vi "Auto Fire.vi"(11 "Run?":bool) -> (3 "Done":bool)   [LabVIEW 2013]
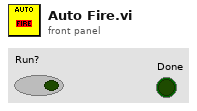
[diagram p1: front panel]
types:
  T1 = typedef "WPI_MotorControlDeviceRef.ctl" = cluster{"DeviceStatus":errorcluster, "Type":enum16{"PWM", "CAN"}, "PWM":cluster{"Digital Module":T2, "PWM Channel":T3, "DeadBand":T4}, "CAN":cluster{"Device Number":u8, "Control Mode":T5, "Semaphore":T6, "Max Vout":dbl}, "Invert":bool, "TransformRef":T7, "InvTransformRef":T7}
  T2 = typedef "FPGA_TypedefDigitalModule.ctl" = enum16{"Digital Module 1", "Digital Module 2"}
  T3 = typedef "FPGA_DIOPWMChannel.ctl" = enum8{"PWM 1", "PWM 2", "PWM 3", "PWM 4", "PWM 5", "PWM 6", "PWM 7", "PWM 8", "PWM 9", "PWM 10", "Invalid"}
  T4 = typedef "WPI_PWMDeadband.ctl" = cluster{"Name":string, "maxPositivePwm":i32, "minPositivePwm":i32, "centerPwm":i32, "maxNegativePwm":i32, "minNegativePwm":i32, "angularRange":u16}
  T5 = typedef "WPI_CANJaguar_ControlMode.ctl" = enum8{"Percent VBus", "Current", "Speed", "Position", "Voltage"}
  T6 = typedef "Semaphore RefNum" = refnum<k1>
  T7 = typedef "WPI_PWMTransform_ConPane.ctl" = refnum<vi>
  T8 = typedef "WPI_DigitalInputDevRef.ctl" = cluster{"DevStatus":errorcluster, "DIO Channel":T9, "Digital Module":T2}
  T9 = typedef "FPGA_DIOChannel.ctl" = enum8{"DIO 1", "DIO 2", "DIO 3", "DIO 4", "DIO 5", "DIO 6", "DIO 7", "DIO 8", "DIO 9", "DIO 10", "DIO 11", "DIO 12", "DIO 13", "DIO 14", "Invalid"}
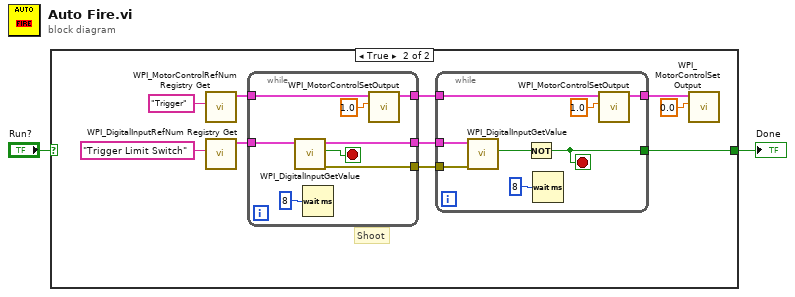
[diagram p0: block diagram]
diagram:
  n1 = case shown="True" "Run?" {
    selector: "Run?" -> [w3 _]
    tunnel: [w3 w4] -> w1
    frame False {
    }
    frame True {
      # "Shoot"
      n2 = call <vilib>:"WPI_MotorControlRefNum Registry Get.vi"("refnum name"="Trigger") -> ("MotorControlDevRef"=w10:T1)  [unwired: 9 in, 1 out]
      n3 = call <vilib>:"WPI_DigitalInputRefNum Registry Get.vi"("refnum name"="Trigger Limit Switch") -> ("DigitalInputDevRef"=w8:T8)  [unwired: 9 in, 1 out]
      n4 = while {
        tunnel: w8 -> [w21]
        tunnel: [w19] -> w5
        tunnel: [w17] -> w6
        tunnel: w10 -> [w15]
        tunnel: [w14] -> w11
        stop <- w20 stop-if-true
        n5 = call <vilib>:"WPI_DigitalInputGetValue.vi"("DigitalInputDevRef"=w21) -> ("error out"=w17:errorcluster, "Value"=w20:bool, "DigitalInputDevRef"=w19:T8)  [unwired: 8 in]
        n6 = Wait (ms)(milliseconds to wait=u32 8) -> ()  [unwired: 1 out]
        n7 = call <vilib>:"WPI_MotorControlSetOutput.vi"("Output"=1.0, "MotorControlDevRef"=w15) -> ("MotorControlDevRef"=w14:T1)  [unwired: 7 in, 2 out]
      }
      n8 = while {
        tunnel: w5 -> [w29]
        tunnel: w6 -> [w26]
        tunnel: w11 -> [w25]
        tunnel: [w23] -> w12
        tunnel: [w22] -> w4
        stop <- w22 stop-if-true
        n9 = call <vilib>:"WPI_DigitalInputGetValue.vi"("error in (no error)"=w26, "DigitalInputDevRef"=w29) -> ("Value"=w28:bool)  [unwired: 7 in, 2 out]
        n10 = Not(x=w28) -> (.not. x?=w22:bool)
        n11 = Wait (ms)(milliseconds to wait=u32 8) -> ()  [unwired: 1 out]
        n12 = call <vilib>:"WPI_MotorControlSetOutput.vi"("Output"=1.0, "MotorControlDevRef"=w25) -> ("MotorControlDevRef"=w23:T1)  [unwired: 7 in, 2 out]
      }
      n13 = call <vilib>:"WPI_MotorControlSetOutput.vi"("Output"=0.0, "MotorControlDevRef"=w12) -> ()  [unwired: 7 in, 3 out]
    }
  }
  "Done" <- w1
